vi "build new output array.vi"(1 "number to insert":dbl, 2 "input array":dbl[](array[numeric])) -> (0 "output array":dbl[](array[numeric]))   [LabVIEW 2012]
doc: "If input array is odd (e.g. for Ch1): inserts the number in last spot of array, combines with original array, and outputs.\nIf input array is even (e.g. for Ch2): outputs original array, with number appended, combined with original array again."
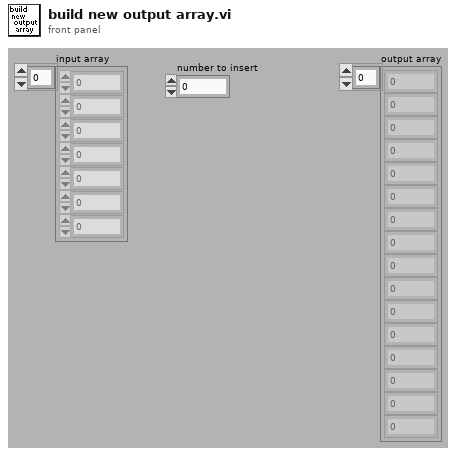
[diagram p1: front panel]
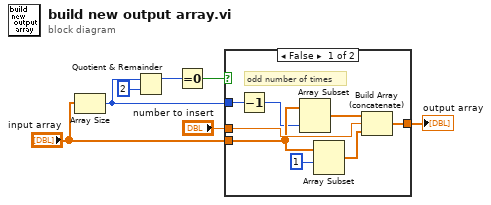
[diagram p0: block diagram]
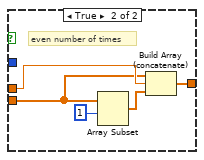
[diagram p2: hidden frame]
diagram:
  n1 = Array Size(array="input array") -> (size(s)=w4:i32)
  n2 = Quotient & Remainder(x=w4, y=i8 2) -> (x-y*floor(x/y)=w6:i32)  [unwired: 1 out]
  n3 = Equal To 0?(x=w6) -> (x = 0?=w5:bool)
  n4 = case shown="False" w5 {
    tunnel: w4 -> [w9 _]
    tunnel: "input array" -> [w10 w18]
    tunnel: "number to insert" -> [w13 w19]
    tunnel: [w12 w20] -> w1
    frame False {
      # "odd number of times"
      n5 = Decrement(x=w9) -> (x-1=w8:i32)
      n6 = Array Subset(array=w10, length=w8) -> (w11:dbl[])  [unwired: 1 in]
      n7 = Array Subset(array=w10, index=1) -> (w14:dbl[])  [unwired: 1 in]
      n8 = Build Array (concatenate)(w11, w13, w14) -> (w12:dbl[])
    }
    frame True {
      # "even number of times"
      n9 = Array Subset(array=w18, index=1) -> (w16:dbl[])  [unwired: 1 in]
      n10 = Build Array (concatenate)(w18, w19, w16) -> (w20:dbl[])
    }
  }
  "output array" <- w1
